vi "Problem1.4.vi"() -> ()   [LabVIEW 2018]
panel:
  out "Edge Change":bool
  out "Edge Off":bool
  out "Edge On":bool
  in  "Boolean\nInput":bool
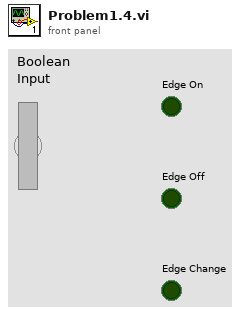
[diagram p1: front panel]
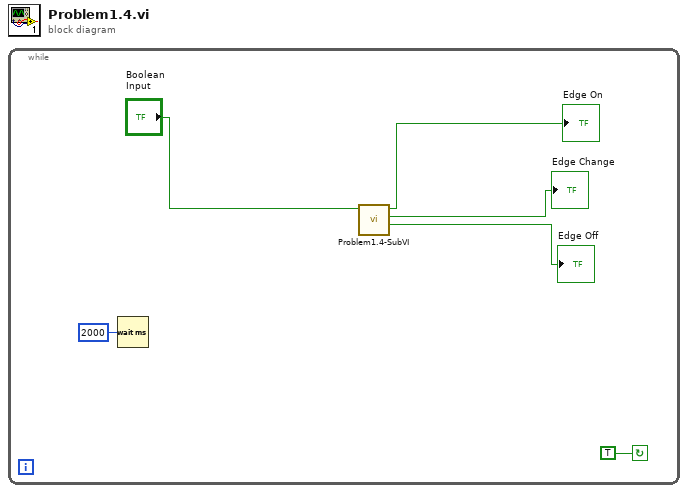
[diagram p0: block diagram]
diagram:
  n1 = while {
    stop <- TRUE continue-if-true
    n2 = Wait (ms)(milliseconds to wait=u32 2000) -> ()  [unwired: 1 out]
    n3 = call "Problem1.4-SubVI.vi"("Boolean\nInput"="Boolean\nInput") -> ("Boolean"=→"Edge Off":bool, "Boolean 3"=→"Edge Change":bool, "Boolean 2"=→"Edge On":bool)  [unwired: 8 in]
  }
